vi "SP Write to INI File.vi"(4 "Step Number":i32=1, 6 "De-Embed Data":bool, 7 "Display":T1={"Lock Control"=FALSE, "Retain Settings"=TRUE, "Formatted Data"=FALSE, "Plot Orientation"=enum."Single", "Plot Controls"=[{"Trace Orientation"=enum."Overlay", "Frequency"={"Change Frequency"=FALSE, "Start"=500.0, "Stop"=1500.0, "Units"=enum."MHz"}, "Markers"=[], "Traces"=[]}, {"Trace Orientation"=enum."Overlay", "Frequency"={"Change Frequency"=FALSE, "Start"=500.0, "Stop"=1500.0, "Units"=enum."MHz"}, "Markers"=[], "Traces"=[]}, {"Trace Orientation"=enum."Overlay", "Frequency"={"Change Frequency"=FALSE, "Start"=500.0, "Stop"=1500.0, "Units"=enum."MHz"}, "Markers"=[], "Traces"=[]}, {"Trace Orientation"=enum."Overlay", "Frequency"={"Change Frequency"=FALSE, "Start"=500.0, "Stop"=1500.0, "Units"=enum."MHz"}, "Markers"=[], "Traces"=[]}]} {"Plot Controls"."Traces"."Reference" format="%#.2g"; "Plot Controls"."Traces"."Display Data" items=["Data", "Memory", "Data/Memory"]; "Plot Controls"."Traces"."Format" items=["Log Mag", "Phase", "Expanded Phase", "Delay", "Smith", "Polar", "Lin Mag", "SWR", "Loss", "Real", "Imaginary"]; "Plot Controls"."Traces"."Scale" min=0.001 step=1.0 format="%#.2g"; "Plot Controls"."Traces"."Position" min=0.0 max=10.0; "Plot Controls"."Frequency"."Stop" format="%.3g"; "Plot Controls"."Frequency"."Start" format="%.3g"}, 8 "error in (no error)":errorcluster, 9 "Requested Stimulus":T9={"Use Instrument Settings"=FALSE, "Blank Frequencies"=FALSE, "Sweep Type"=enum."Linear", "Sweep"={"Fstart"=500.0, "Fstop"=1500.0, "Units"=enum."MHz", "Points"=201}, "Power (dBm)"=999.0, "IFBW (Hz)"=-1.0, "Sweep Time (s)"=-1.0, "Calibration"={"State"=FALSE, "String"=""}} {"Sweep Time (s)" format="%.3g"}, 10 "Parameters to Measure":T11[](array[typedef]) {"Channel" min=1 max=99 step=1; "Parameter"."Stimulus Port" min=1 step=1; "Parameter"."Response Port" min=1 step=1}, 11 "Data to Write":enum16{"Calibration", "Display", "De-Embed"}(ring)) -> (0 "error out":errorcluster)   [LabVIEW 2011]
uses:
  TypeDefs/SP Parameter to Measure.ctl
  TypeDefs/SP Parameter.ctl
  TypeDefs/SP Calibration State.ctl
  TypeDefs/SP Measurement Format.ctl
  TypeDefs/SP Stimulus Parameters.ctl
  TypeDefs/SP Frequency Units.ctl
  TypeDefs/SP Display Parameters.ctl
  TypeDefs/SP Display Plot Controls Cluster.ctl
  TypeDefs/SP Marker Cluster.ctl
  TypeDefs/SP Marker Type.ctl
  TypeDefs/SP Display Trace Controls.ctl
  TypeDefs/SP Display Format.ctl
  TypeDefs/SP Display Data.ctl
  <vilib>/Utility/config.llb/Write Key (String).vi
  <vilib>/Utility/config.llb/NI_LVConfig.lvlib
panel:
  # "Div"
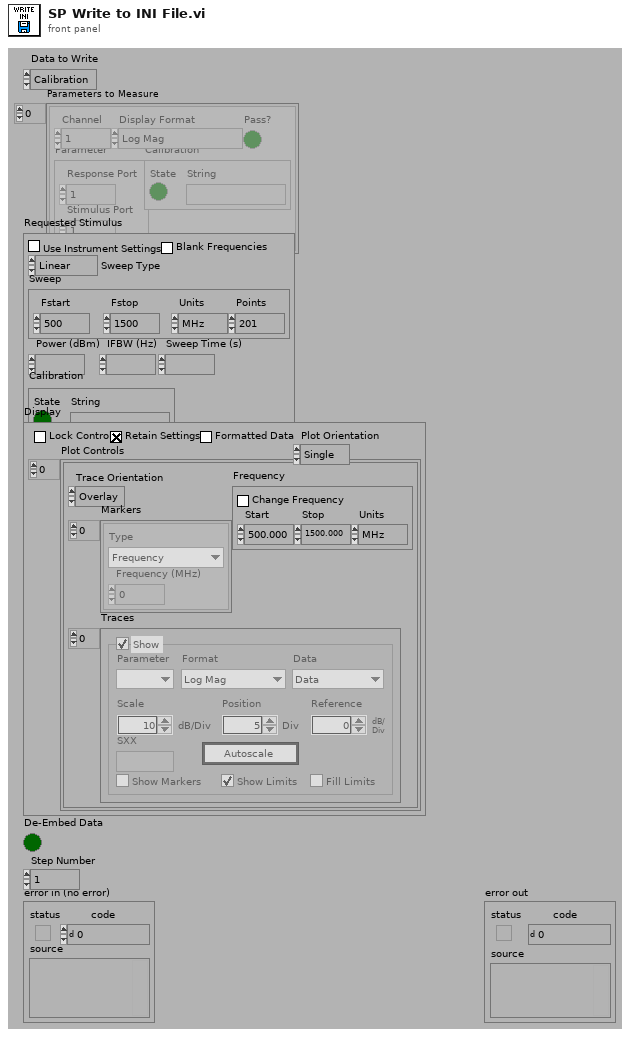
[diagram p1: front panel]
types:
  T1 = typedef "SP Display Parameters.ctl" = cluster{"Lock Control":bool, "Retain Settings":bool, "Formatted Data":bool, "Plot Orientation":enum32{"Single", "Dual", "Quad"}, "Plot Controls":T2[]}
  T2 = typedef "SP Display Plot Controls Cluster.ctl" = cluster{"Trace Orientation":enum32{"Overlay", "Split"}, "Frequency":cluster{"Change Frequency":bool, "Start":dbl, "Stop":dbl, "Units":T3}, "Markers":T4[], "Traces":T6[]}
  T3 = typedef "SP Frequency Units.ctl" = enum16{"Hz", "kHz", "MHz", "GHz", "Points"}
  T4 = typedef "SP Marker Cluster.ctl" = cluster{"Type":T5, "Frequency (MHz)":dbl}
  T5 = typedef "SP Marker Type.ctl" = enum16{"Frequency", "Trace Maximum", "Trace Minimum", "Limit Maximum", "Limit Minimum"}
  T6 = typedef "SP Display Trace Controls.ctl" = cluster{"Trace On":bool, "Measure":i32, "Format":T7, "Autoscale":bool, "Reference":dbl, "\nRefUnit":string, "Position":dbl, "Scale":dbl, "ScaleUnit":string, "LimitOn":bool, "LimitFill":bool, "Display Data":T8, "Show Markers":bool, "SXX":string}
  T7 = typedef "SP Display Format.ctl" = i32
  T8 = typedef "SP Display Data.ctl" = u16
  T9 = typedef "SP Stimulus Parameters.ctl" = cluster{"Use Instrument Settings":bool, "Blank Frequencies":bool, "Sweep Type":enum32{"Linear", "Logarithmic", "List", "Power", "CW"}, "Sweep":cluster{"Fstart":dbl, "Fstop":dbl, "Units":T3, "Points":i32}, "Power (dBm)":dbl, "IFBW (Hz)":dbl, "Sweep Time (s)":dbl, "Calibration":T10}
  T10 = typedef "SP Calibration State.ctl" = cluster{"State":bool, "String":string}
  T11 = typedef "SP Parameter to Measure.ctl" = cluster{"Channel":i8, "Parameter":T12, "Calibration":T10, "Display Format":T13, "Pass?":bool}
  T12 = typedef "SP Parameter.ctl" = cluster{"Stimulus Port":i8, "Response Port":i8}
  T13 = typedef "SP Measurement Format.ctl" = enum32{"Log Mag", "Phase", "Delay", "Smith (R+jX)", "Polar (Re/Im)", "Linear Mag", "SWR", "Real", "Imaginary", "Smith (Lin/Phase)", "Smith (Log/Phase)", "Smith (Real/Imag)", "Smith (G+jB)", "Polar (Lin/Phase)", "Polar (Log/Phase)", "Expanded Phase", "Positive Phase", "Inverted Smith", "Unwrapped Phase", "Power Out", "Power In", "Linear Mag/Phase", "Log Mag/Phase", "Real/Imaginary"}
  T14 = typedef "NI_LVConfig.lvlib/Config Data RefNum.ctl" = refnum<k1>
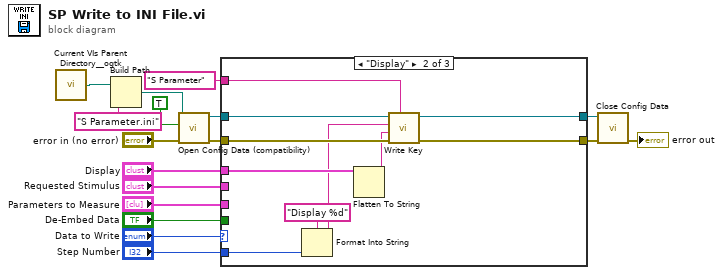
[diagram p0: block diagram]
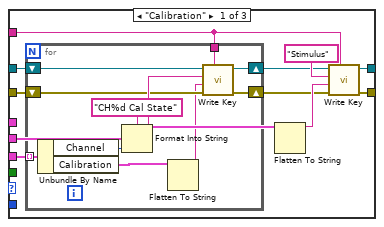
[diagram p2: hidden frame]
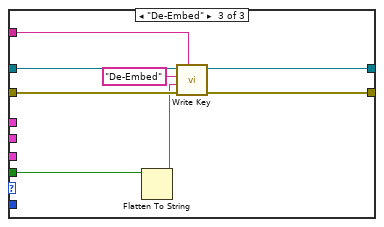
[diagram p3: hidden frame]
diagram:
  n1 = call "Current VIs Parent Directory__ogtk.vi"() -> ("Parent Directory (+ Relative)"=w1:path)  [unwired: 5 in]
  n2 = Build Path(base path=w1, name or relative path="S Parameter.ini") -> (appended path=w4:path)
  n3 = call <vilib>:"Open Config Data (compatibility).vi"("error in (no error)"="error in (no error)", "create file if necessary (T)"=TRUE ("create file if necessary? (T)"), "configuration file path"=w4) -> ("error out"=w11:errorcluster, "refnum"=w10:T14)  [unwired: 6 in, 1 out]
  n4 = case shown="\"Display\"" "Data to Write" {
    tunnel: [w27 w44 w53] -> w15
    tunnel: [w26 w45 w54] -> w14
    tunnel: w11 -> [w23 w49 w57]
    tunnel: w10 -> [w22 w48 w56]
    tunnel: "Parameters to Measure" -> [w19 _ _]
    tunnel: "Requested Stimulus" -> [w24 _ _]
    tunnel: "S Parameter" ("section") -> [w18 w47 w55]
    tunnel: "Display" -> [_ w46 _]
    tunnel: "De-Embed Data" -> [_ _ w50]
    tunnel: "Step Number" -> [_ w42 _]
    frame "Calibration" {
      n5 = for {
        tunnel: w19 -> [w38] mode=indexing
        shift-right: [w35] -> w20
        shift-left: w23 -> [w36]
        shift-right: [w34] -> w21
        shift-left: w22 -> [w33]
        tunnel: w18 -> [w32]
        n6 = Unbundle By Name(w38) -> ("Channel"=w29:i8, "Calibration"=w31:T10)
        n7 = Format Into String(format string="CH%d Cal State", w29) -> (resulting string=w37:string)  [unwired: 2 in, 1 out]
        n8 = Flatten To String(anything=w31) -> (data string=w30:string)  [unwired: 1 in, 4 out]
        n9 = call-poly <vilib>:"Write Key.vi"("section"=w32, "error in (no error)"=w36, "value"=w30, "key"=w37, "refnum"=w33) -> ("error out"=w35:errorcluster, "refnum out"=w34:T14)  [unwired: 1 in, 4 out]
      }
      n10 = Flatten To String(anything=w24) -> (data string=w28:string)  [unwired: 1 in, 4 out]
      n11 = call-poly <vilib>:"Write Key.vi"("section"=w18, "error in (no error)"=w20, "value"=w28, "key"="Stimulus", "refnum"=w21) -> ("error out"=w26:errorcluster, "refnum out"=w27:T14)  [unwired: 1 in, 4 out]
    }
    frame "Display" {
      n12 = Format Into String(format string="Display %d" ("section"), w42) -> (resulting string=w40:string)  [unwired: 2 in, 1 out]
      n13 = Flatten To String(anything=w46) -> (data string=w43:string)  [unwired: 1 in, 4 out]
      n14 = call-poly <vilib>:"Write Key.vi"("section"=w47, "error in (no error)"=w49, "value"=w43, "key"=w40, "refnum"=w48) -> ("error out"=w45:errorcluster, "refnum out"=w44:T14)  [unwired: 1 in, 4 out]
    }
    frame "De-Embed" {
      n15 = Flatten To String(anything=w50) -> (data string=w52:string)  [unwired: 1 in, 4 out]
      n16 = call-poly <vilib>:"Write Key.vi"("section"=w55, "error in (no error)"=w57, "value"=w52, "key"="De-Embed" ("section"), "refnum"=w56) -> ("error out"=w54:errorcluster, "refnum out"=w53:T14)  [unwired: 1 in, 4 out]
    }
  }
  n17 = call <vilib>:"Close Config Data.vi"("error in (no error)"=w14, "refnum"=w15) -> ("error out"=→"error out":errorcluster)  [unwired: 1 in, 8 out]
